vi "SftpGetState.vi"(0 "error in":errorcluster, 11 "Sftp":refnum<k24>) -> (4 "error out":errorcluster, 15 "Connected":bool)   [LabVIEW 2022 SP3, in "UnderAutomation.UniversalRobots.lvlib"]
uses:
  UnderAutomation.UniversalRobots.lvlib
  C:/Users/fg/Documents/UniversalRobots.vi/LabVIEW_2024/UnderAutomation.UniversalRobots/lib/UnderAutomation.UniversalRobots.dll
  LabVIEW_2024/UnderAutomation.UniversalRobots/lib/UnderAutomation.UniversalRobots.dll
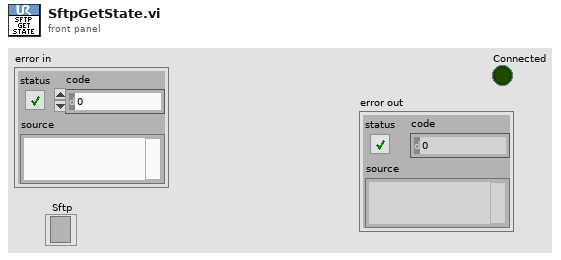
[diagram p1: front panel]
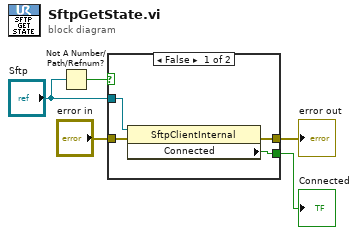
[diagram p0: block diagram]
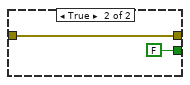
[diagram p2: hidden frame]
diagram:
  n1 = Not A Number/Path/Refnum?(number/path/refnum="Sftp") -> (NaN/Path/Refnum?=w1:bool)
  n2 = case shown="False" w1 {
    tunnel: [w9 FALSE ("Connected")] -> w5
    tunnel: [w8 w11] -> w4
    tunnel: "error in" -> [w7 w11]
    tunnel: "Sftp" -> [w6 _]
    frame False {
      n3 = property class="SftpClientInternal"(reference=w6, error in=w7) -> (error out=w8:errorcluster, "Connected"=w9:bool)  [unwired: 1 out]
    }
    frame True {
    }
  }
  "error out" <- w4
  "Connected" <- w5
